vi "Abort.vi"(8 "error in (no error)":errorcluster, 11 "DAQmx Base in":refnum<class "NI DAQmx Base.lvclass">) -> (0 "error out":errorcluster, 3 "DAQmx Base out":refnum<class "NI DAQmx Base.lvclass">)   [LabVIEW 2020, in "NI DAQmx.lvlib" / "NI DAQmx Base.lvclass"]
uses:
  NI DAQmx Base.lvclass
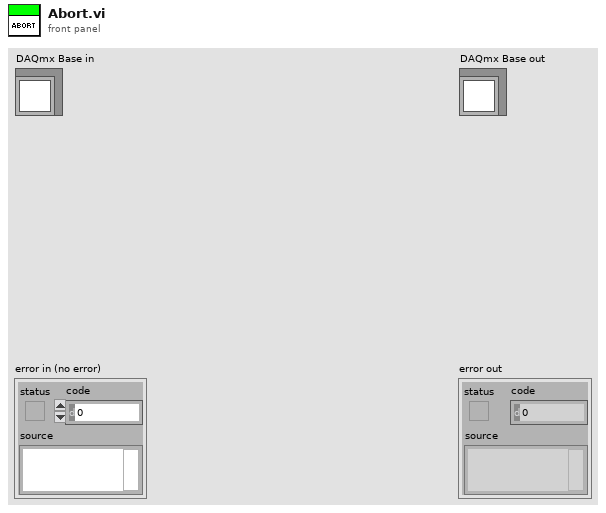
[diagram p1: front panel]
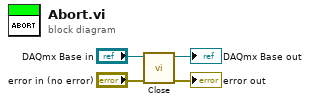
[diagram p0: block diagram]
diagram:
  n1 = call-dynamic "Close.vi"("error in (no error)"="error in (no error)", "DAQmx Base in"="DAQmx Base in") -> ("error out"=→"error out":errorcluster, "DAQmx Base out"=→"DAQmx Base out":refnum<class "NI DAQmx Base.lvclass">)  [unwired: 8 in]
